vi "Flock_Shared_Initialize Queue.vi"(8 "Error In":errorcluster) -> (0 "error out":errorcluster)   [LabVIEW 2013, in "Flock_Shared_Messaging.lvlib" / "Flock_Shared_CentralProcessMessaging.lvlib"]
uses:
  Flock_Shared_CentralProcessMessaging.lvlib
  FGV_Action.ctl
  Flock_Shared_Messaging.lvlib
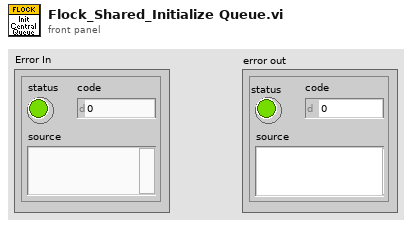
[diagram p1: front panel]
types:
  T1 = typedef "FGV_Action.ctl" = enum16{"Initalize Central", "Initialize Local", "Get", "Delete Local"}
  T2 = typedef "AMC.lvlib/Message Queue.ctl" = refnum<queue>
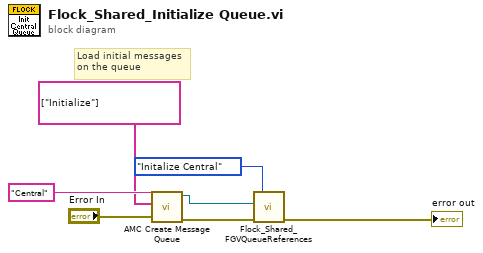
[diagram p0: block diagram]
diagram:
  # "Load initial messages\non the queue"
  n1 = call <vilib>:"AMC Create Message Queue.vi"("error in (no error)"="Error In", "Initial Message Names"=string[] ["Initialize"], "Message Queue Name"="Central") -> ("error out"=w3:errorcluster, "Message Queue out"=w4:T2)  [unwired: 1 in, 6 out]
  n2 = call "Flock_Shared_FGVQueueReferences.vi"("Action"=FGV_Action."Initalize Central", "error in (no error)"=w3, "Central Queue in"=w4) -> ("error out"=→"error out":errorcluster)  [unwired: 6 in, 2 out]
